vi "Globals.vi"(7 "action":T9, 8 "error in":errorcluster, 10 "Data Display Params":T1, 11 "Data Acquisition":T3={"Experiment Type"=enum."PID Sample", "Experiment Name"="", "Operator Name"="", "Notes"="", "TDMS File Path"=path "", "Data Acquisition State"=FALSE, "PID Voltage Sweep"={"Voltage Step (V)"=1.0, "Voltage Range (V)"={10, 20}, "Time Step (s)"=5.0, "Voltage Step Direction"=enum."Low 2 High"}, "MFC Challenge Profile - Heaviside Step"={"Valve Open Duration"=20, "MFC Flow Rate"=100.0, "Valve Open Repeats"=50, "Valve Open Start"=1}, "MFC Challenge Profile"=enum."Heaviside", "MFC Challenge Profile - Staircase"={"Step Time Duration"=1, "Step Flow Rate"=0.0, "Steps"=1, "Valve Open Start"=1, "Recovery"=FALSE, "Repeats"=1}} {"MFC Challenge Profile - Staircase"."Repeats" min=1 max=1000 step=1; "MFC Challenge Profile - Staircase"."Valve Open Start" min=1 max=1000 step=1; "MFC Challenge Profile - Staircase"."Steps" min=1 max=1000 step=1; "MFC Challenge Profile - Staircase"."Step Flow Rate" min=0.0 max=200.0 scale=0.0..200.0; "MFC Challenge Profile - Staircase"."Step Time Duration" min=1 max=1000 step=1; "MFC Challenge Profile - Heaviside Step"."Valve Open Start" min=1 max=1000 step=1; "MFC Challenge Profile - Heaviside Step"."Valve Open Repeats" min=1 max=1000 step=1; "MFC Challenge Profile - Heaviside Step"."MFC Flow Rate" min=0.0 max=200.0 scale=0.0..200.0; "MFC Challenge Profile - Heaviside Step"."Valve Open Duration" min=1 max=1000 step=1; "PID Voltage Sweep"."Voltage Range (V)" scale=0.0..500.0}) -> (0 "error out":errorcluster, 2 "Data Display Params":T1, 3 "Data Acquisition":T3={"Experiment Type"=enum."PID Sample", "Experiment Name"="", "Operator Name"="", "Notes"="", "TDMS File Path"=path "", "Data Acquisition State"=FALSE, "PID Voltage Sweep"={"Voltage Step (V)"=1.0, "Voltage Range (V)"={10, 20}, "Time Step (s)"=5.0, "Voltage Step Direction"=enum."Low 2 High"}, "MFC Challenge Profile - Heaviside Step"={"Valve Open Duration"=20, "MFC Flow Rate"=100.0, "Valve Open Repeats"=50, "Valve Open Start"=1}, "MFC Challenge Profile"=enum."Heaviside", "MFC Challenge Profile - Staircase"={"Step Time Duration"=1, "Step Flow Rate"=0.0, "Steps"=1, "Valve Open Start"=1, "Recovery"=FALSE, "Repeats"=1}} {"MFC Challenge Profile - Staircase"."Repeats" min=1 max=1000 step=1; "MFC Challenge Profile - Staircase"."Valve Open Start" min=1 max=1000 step=1; "MFC Challenge Profile - Staircase"."Steps" min=1 max=1000 step=1; "MFC Challenge Profile - Staircase"."Step Flow Rate" min=0.0 max=200.0 scale=0.0..200.0; "MFC Challenge Profile - Staircase"."Step Time Duration" min=1 max=1000 step=1; "MFC Challenge Profile - Heaviside Step"."Valve Open Start" min=1 max=1000 step=1; "MFC Challenge Profile - Heaviside Step"."Valve Open Repeats" min=1 max=1000 step=1; "MFC Challenge Profile - Heaviside Step"."MFC Flow Rate" min=0.0 max=200.0 scale=0.0..200.0; "MFC Challenge Profile - Heaviside Step"."Valve Open Duration" min=1 max=1000 step=1; "PID Voltage Sweep"."Voltage Range (V)" scale=0.0..500.0})   [LabVIEW 2011]
uses:
  Globals.ctl
  Controls/Data Acquisition Parameters.ctl
  Controls/DAQ Type.ctl
  Controls/PID Voltage Seep Settings.ctl
  Controls/MFC Challenge Profile - Heaviside Step.ctl
  Controls/MFC Challen Profile Type.ctl
  Controls/MFC Challenge Profile - Staircase.ctl
  Controls/Data Display Parameters.ctl
  Controls/Display Mode.ctl
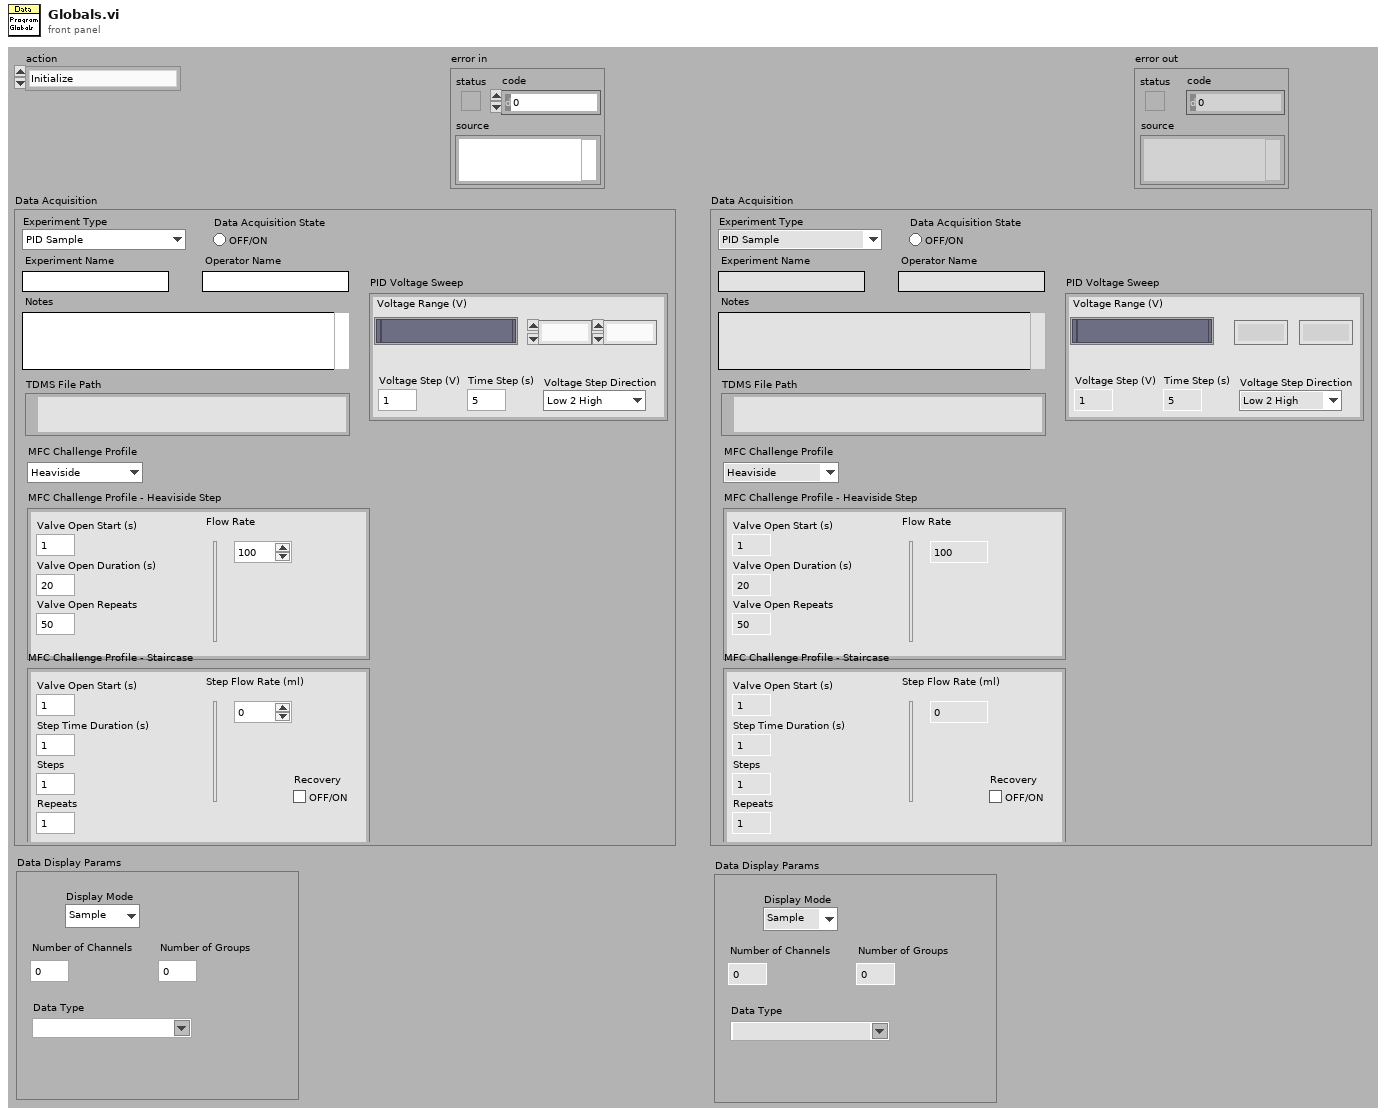
[diagram p1: front panel]
types:
  T1 = typedef "Data Display Parameters.ctl" = cluster{"Number of Channels":u32, "Number of Groups":u32, "Display Mode":T2, "Data Type":string}
  T2 = typedef "Display Mode.ctl" = enum16{"Sample", "Run"}
  T3 = typedef "Data Acquisition Parameters.ctl" = cluster{"Experiment Type":T4, "Experiment Name":string, "Operator Name":string, "Notes":string, "TDMS File Path":path, "Data Acquisition State":bool, "PID Voltage Sweep":T5, "MFC Challenge Profile - Heaviside Step":T6, "MFC Challenge Profile":T7, "MFC Challenge Profile - Staircase":T8}
  T4 = typedef "DAQ Type.ctl" = enum16{"PID Sample", "PID with PS Challenge", "PID with MFC Challenge", "Multimeter Sample", "Multimeter with MFC Challenge"}
  T5 = typedef "PID Voltage Seep Settings.ctl" = cluster{"Voltage Step (V)":dbl, "Voltage Range (V)":cluster{u16, u16}, "Time Step (s)":dbl, "Voltage Step Direction":enum16{"High 2 Low", "Low 2 High"}}
  T6 = typedef "MFC Challenge Profile - Heaviside Step.ctl" = cluster{"Valve Open Duration":u16, "MFC Flow Rate":dbl, "Valve Open Repeats":u16, "Valve Open Start":u16}
  T7 = typedef "MFC Challen Profile Type.ctl" = enum16{"Heaviside", "Staircase"}
  T8 = typedef "MFC Challenge Profile - Staircase.ctl" = cluster{"Step Time Duration":u16, "Step Flow Rate":dbl, "Steps":u16, "Valve Open Start":u16, "Recovery":bool, "Repeats":u16}
  T9 = typedef "Globals.ctl" = enum16{"Initialize", "Get DAQ Params", "Get Data Display Params", "Set DAQ Params", "Set Data Display Params"}
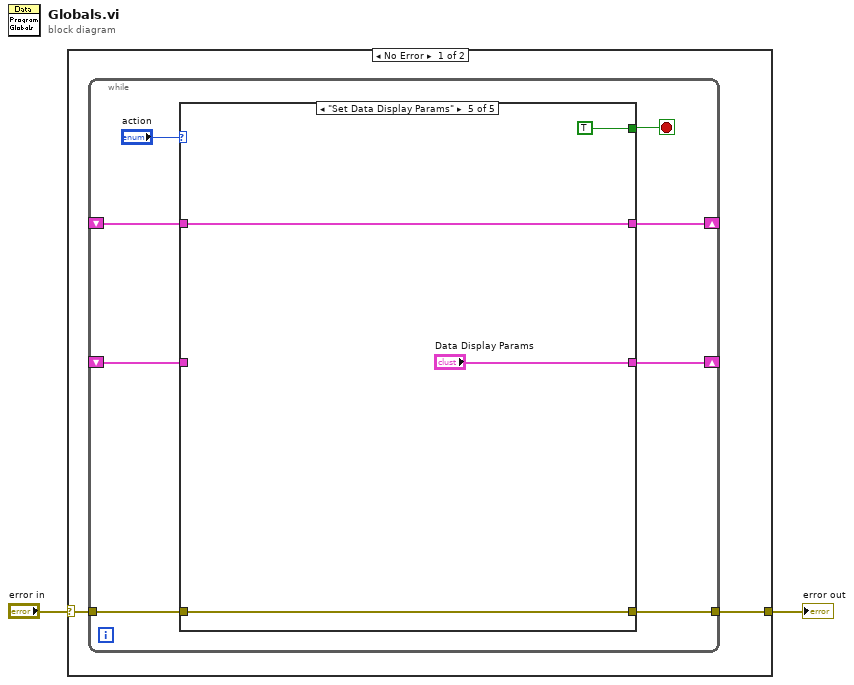
[diagram p0: block diagram]
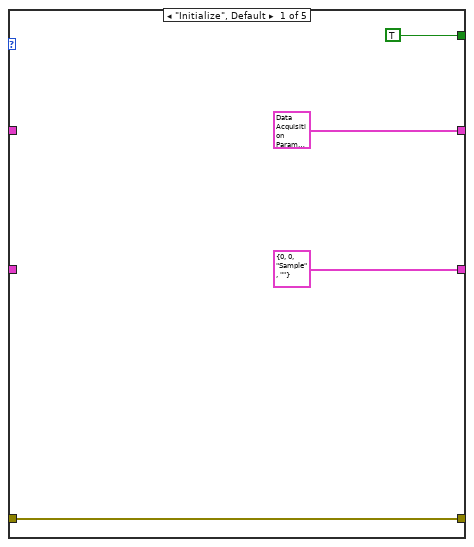
[diagram p2: hidden frame]
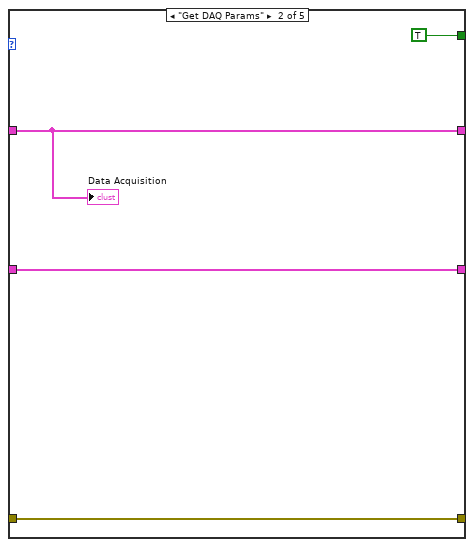
[diagram p3: hidden frame]
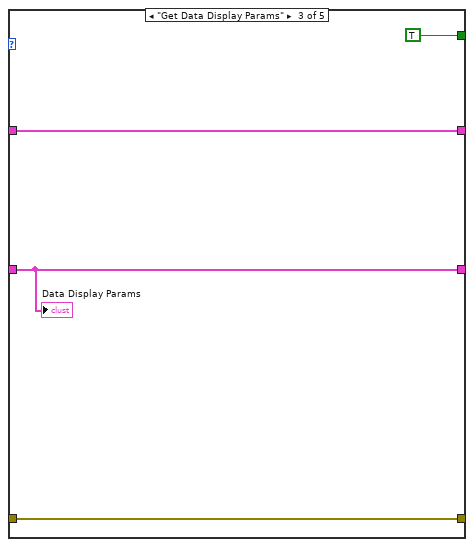
[diagram p4: hidden frame]
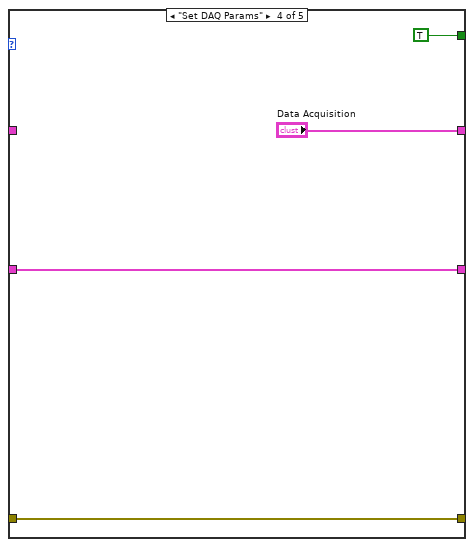
[diagram p5: hidden frame]
diagram:
  n1 = case shown="No Error" "error in" {
    selector: "error in" -> [w4 w33]
    tunnel: [w3 w33] -> w1
    frame No Error {
      n2 = while {
        tunnel: w4 -> [w11]
        tunnel: [w10] -> w3
        shift-right: [w8] -> _
        shift-left: _ -> [w7]
        shift-right: [w6] -> _
        shift-left: _ -> [w5]
        stop <- w9 stop-if-true
        n3 = case shown="\"Set Data Display Params\"" "action" {
          tunnel: w11 -> [w16 w20 w21 w28 w29]
          tunnel: [w16 w20 w21 w28 w29] -> w10
          tunnel: [TRUE TRUE TRUE TRUE TRUE] -> w9
          tunnel: [T3 {"Experiment Type"=enum."PID Sample", "Experiment Name"="", "Operator Name"="", "Notes"="", "TDMS File Path"=path "", "Data Acquisition State"=FALSE, "PID Voltage Sweep"={"Voltage Step (V)"=0.0, "Voltage Range (V)"={0, 0}, "Time Step (s)"=0.0, "Voltage Step Direction"=enum."High 2 Low"}, "MFC Challenge Profile - Heaviside Step"={"Valve Open Duration"=0, "MFC Flow Rate"=0.0, "Valve Open Repeats"=0, "Valve Open Start"=0}, "MFC Challenge Profile"=enum."Heaviside", "MFC Challenge Profile - Staircase"={"Step Time Duration"=0, "Step Flow Rate"=0.0, "Steps"=0, "Valve Open Start"=0, "Recovery"=FALSE, "Repeats"=0}} ("Data Acquisition") w18 w24 "Data Acquisition" w32] -> w8
          tunnel: w7 -> [_ w18 w24 _ w32]
          tunnel: [T1 {"Number of Channels"=0, "Number of Groups"=0, "Display Mode"=enum."Sample", "Data Type"=""} ("Data Display Params") w17 w23 w25 "Data Display Params"] -> w6
          tunnel: w5 -> [_ w17 w23 w25 _]
          frame "Initialize", Default {
          }
          frame "Get DAQ Params" {
            "Data Acquisition" <- w18
          }
          frame "Get Data Display Params" {
            "Data Display Params" <- w23
          }
          frame "Set DAQ Params" {
          }
          frame "Set Data Display Params" {
          }
        }
      }
    }
    frame Error {
    }
  }
  "error out" <- w1
